vi "histCase.vi"(0 "CaseControl":T2, 1 "present case":T1, 3 "event":T1, 6 "finish?":bool=TRUE, 8 "retry":i32) -> (14 "CaseControl":T2, 17 "event":T1)   [LabVIEW 2018]
uses:
  TEST/Typedefs/Command.ctl
  Typedefs/CaseControl.ctl
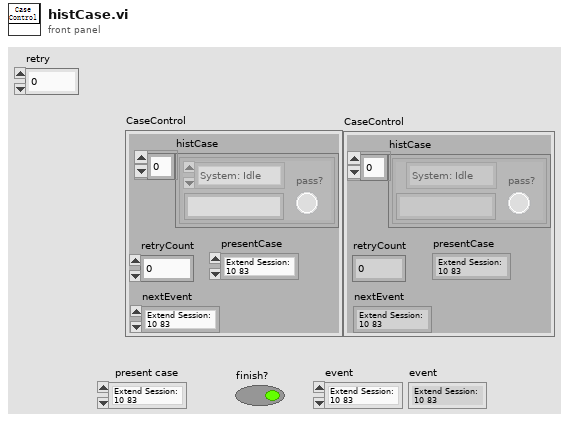
[diagram p1: front panel]
types:
  T1 = typedef "Command.ctl" = enum16{"Extend Session: 10 83", "Tester Present: 3E 80", "Resquest Seed: 27 01", "Send Key: 27 02", "Check FBL:  31 01 FD 02", "Control DTC: 85 82", "Comm Control: 28 83 01", "Program Session Request: 10 02", "Request Seed: 27 35", "Seed Key: 27 36", "Request Download: 34 00 44", "Transfer Data: 36 XX YY", "More Data?", "Request Transfer Exit: 37", "Check Flash Driver Validity: 01 FD 03", "More Segment?", "Write Data Fingereint: 23 F1 F0+26", "EraseFlashMemory Routine: 31 01 FD 00 44", "More segment?(each file)", "CheckAppSwAppData Validity: 31 01 FD 04 44", "CheckAppSwAppData Dependency: 31 01 fd 01", "ECU Reset: 11 81", "System: Init", "System: Idle", "System: Error", "System: Wait", "System: Delay", "System: CAN Send 1", "System: CAN Send 2", "System: CAN Read", "System: Exit"}
  T2 = typedef "CaseControl.ctl" = cluster{"histCase":cluster{"time":string, "event":T1, "pass?":bool}[], "retryCount":i32, "presentCase":T1, "nextEvent":T1}
  T3 = cluster{"time":string, "event":T1, "pass?":bool}[]
  T4 = cluster{"time_YMD":string, "  present case":T1, "finish?":bool}
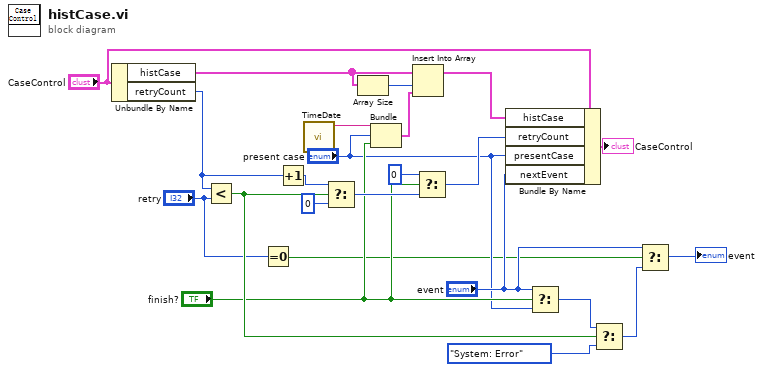
[diagram p0: block diagram]
diagram:
  n1 = Unbundle By Name("CaseControl") -> ("histCase"=w22:T3, "retryCount"=w18:i32)
  n2 = Less?(x=w18, y="retry") -> (x < y?=w17:bool)
  n3 = Equal To 0?(x="retry") -> (x = 0?=w2:bool)
  n4 = Increment(x=w18) -> (x+1=w15:i32)
  n5 = call "TimeDate.vi"() -> ("time_YMD"=w9:string)  [unwired: 10 in, 1 out]
  n6 = Select(t=w15, s=w17, f=0 ("t")) -> (s? t:f=w13:i32)
  n7 = Array Size(array=w22) -> (size(s)=w23:i32)
  n8 = Bundle("time_YMD"=w9, "present case"="present case", "finish?"="finish?") -> (w10:T4)  [unwired: 1 in]
  n9 = Insert Into Array(array=w22, index=w23, new element=w10) -> (w20:T3)
  n10 = Select(t=0, s="finish?", f=w13) -> (s? t:f=w11:i32)
  n11 = Bundle By Name(cluster="CaseControl", "histCase"=w20, "retryCount"=w11, "presentCase"="present case", "nextEvent"="event") -> (→"CaseControl":T2)
  n12 = Select(t="event", s="finish?", f="present case") -> (s? t:f=w14:T1)
  n13 = Select(t=w14, s=w17, f=Command."System: Error") -> (s? t:f=w5:T1)
  n14 = Select(t="event", s=w2, f=w5) -> (s? t:f=→"event":T1)
